vi "CWConvolution.vi"(0 "delay waveform":dbl[](array[numeric])=[0.0] format="%.2f", 1 "Boolean":bool, 2 "delay pts":i32, 3 "h(r,t)":dbl[](array[numeric]) format="%.2f", 4 "Variables":T1={"Number of rings"=8, "sound spd (cm/s)"=150000, "z span (cm)"=8.0, "z steps"=20, "y span (cm)"=0.2, "y steps"=20, "time step (s)"=1e-08, "z"=0.0, "y"=0.0, "ref delay"=0.0, "freq (MHz)"=4.71, "cycles"=300} {"freq (MHz)" format="%.2f"; "z span (cm)" format="%.2f"; "y" format="%.2f"; "ref delay" format="%.2f"; "y span (cm)" format="%.3f"; "z" format="%.2f"; "time step (s)" format="%.2e"}) -> (5 "X*Y":dbl[](array[numeric]) format="%.2f", 7 "pre-zeros":i32)   [LabVIEW 2022 SP3]
uses:
  <vilib>/Analysis/2dsp.llb/Real FFT.vi
  <vilib>/Analysis/2dsp.llb/Inverse Complex FFT.vi
  <vilib>/Analysis/2dsp.llb/1D Convolution (DBL).vi
  <vilib>/measure/NI_MABase.lvlib
  <vilib>/Analysis/NI_AALPro.lvlib
panel:
  in  "Case Constant\n(See Context Help)":bool
  out "Waveform Graph 2":dbl[](graph)
  out "Waveform Graph":dbl[](graph)
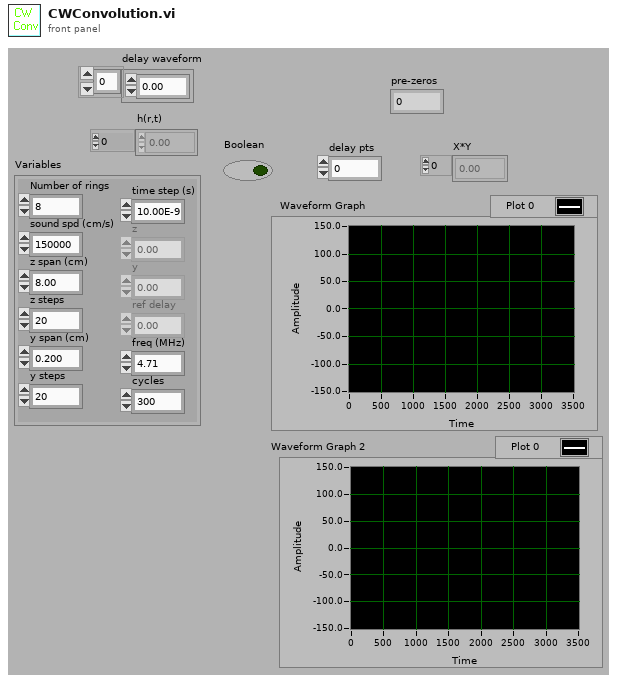
[diagram p1: front panel]
types:
  T1 = cluster{"Number of rings":i32, "sound spd (cm/s)":i32, "z span (cm)":dbl, "z steps":i32, "y span (cm)":dbl, "y steps":i32, "time step (s)":sgl, "z":dbl, "y":dbl, "ref delay":dbl, "freq (MHz)":dbl, "cycles":i32}
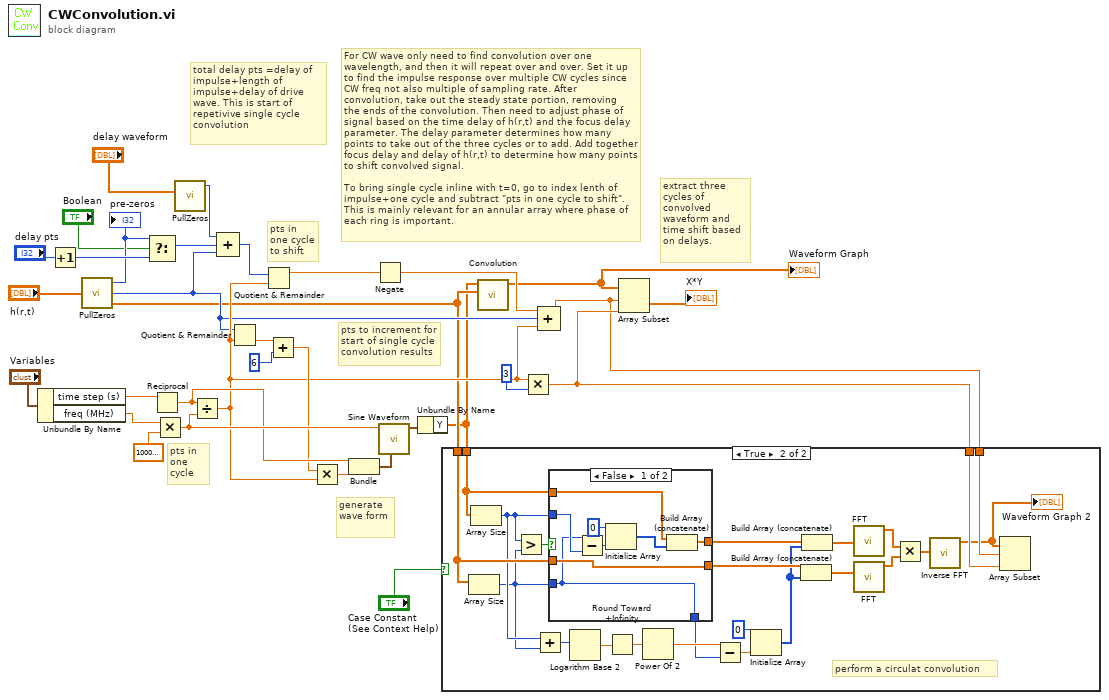
[diagram p0: block diagram]
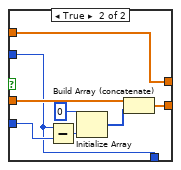
[diagram p3: hidden frame]
diagram:
  # "pts to increment for start of single cycle convolution results"
  # "extract three cycles of convolved waveform and time shift based on delays."
  # "generate wave form"
  # "pts in one cycle"
  # "pts in one cycle to shift"
  # "total delay pts =delay of impulse+length of impulse+delay of drive wave. This is start of repetivive single cycle convolution"
  # "For CW wave only need to find convolution over one wavelength, and then it will repeat over and over. Set it up to find the impulse response over multiple CW cycles since CW freq not also multiple of sampling rate. After convolution, take out the steady state portion, removing  the ends of the convolution. Then need to adjust phase of signal based on the time delay of h(r,t) and the focus delay parameter. The delay parameter determines how many points to take out of the three cycles or to add. Add together focus delay and delay of h(r,t) to determine how many points to shift convolved signal.\n\nTo bring single cycle inline with t=0, go to index lenth of impulse+one cycle and subtract \"pts in one cycle to shift\". This is mainly relevant for an annular array where phase of each ring is important."
  n1 = Unbundle By Name("Variables") -> ("time step (s)"=w22:sgl, "freq (MHz)"=w31:dbl)
  n2 = Increment(x="delay pts") -> (x+1=w10:i32)
  n3 = call "PullZeros.vi"("input"="h(r,t)") -> ("output"=w7:dbl[], "non zero points"=w16:i32, "pre-zeros"=w9:i32)  [unwired: 2 out]
  "pre-zeros" <- w9
  n4 = Select(t=w9, s="Boolean", f=w10) -> (s? t:f=w13:i32)
  n5 = Reciprocal(x=w22) -> (1/x=w28:sgl)
  n6 = Multiply(x=w31, y=1000000.0) -> (x*y=w29:dbl)
  n7 = call "PullZeros.vi"("input"="delay waveform") -> ("pre-zeros"=w17:i32)  [unwired: 4 out]
  n8 = Divide(x=w28, y=w29) -> (x/y=w20:dbl)
  n9 = Compound Arithmetic op=ADD(w17, w13, w16) -> (w15:i32)
  n10 = Quotient & Remainder(x=w16, y=w20) -> (floor(x/y)=w21:dbl)  [unwired: 1 out]
  n11 = Quotient & Remainder(x=w15, y=w20) -> (x-y*floor(x/y)=w19:dbl)  [unwired: 1 out]
  n12 = Add(x=w21, y=6) -> (x+y=w25:dbl)
  n13 = Multiply(x=w25, y=w20) -> (x*y=w27:dbl)
  n14 = Bundle(w28, w27) -> (w32:cluster{sgl, dbl})  [unwired: 1 out]
  n15 = Negate(x=w19) -> (-x=w14:dbl)
  n16 = call <vilib>:"Sine Waveform.vi"("sampling info"=w32, "frequency"=w29) -> ("signal out"=w26:waveform(dbl))  [unwired: 5 in, 4 out]
  n17 = Unbundle By Name(w26) -> ("Y"=w6:dbl[])
  n18 = call-poly <vilib>:"Convolution.vi"("Y"=w7, "X"=w6) -> ("X * Y"=w2:dbl[])  [unwired: 1 in, 8 out]
  "Waveform Graph" <- w2
  n19 = Multiply(x=w20, y=3) -> (x*y=w5:dbl)
  n20 = Compound Arithmetic op=ADD(w14, w16, w20) -> (w4:dbl)
  n21 = case shown="True" "Case Constant\n(See Context Help)" {
    tunnel: w7 -> [_ w52]
    tunnel: w6 -> [_ w51]
    tunnel: w5 -> [_ w50]
    tunnel: w4 -> [_ w49]
    frame False {
    }
    frame True {
      # "perform a circulat convolution"
      n22 = Array Size(array=w52) -> (size(s)=w47:i32)
      n23 = Array Size(array=w51) -> (size(s)=w48:i32)
      n24 = Greater?(x=w48, y=w47) -> (0:w53:bool)
      n25 = Add(x=w48, y=w47) -> (x+y=w46:i32)
      n26 = case shown="False" w53 {
        tunnel: w48 -> [w60 w65]
        tunnel: w47 -> [w57 w72]
        tunnel: w52 -> [w58 w69]
        tunnel: [w58 w67] -> w41
        tunnel: w51 -> [w61 w66]
        tunnel: [w59 w66] -> w40
        tunnel: [w57 w65] -> w37
        frame False {
          n27 = Subtract(x=w57, y=w60) -> (x-y=w63:i32)
          n28 = Initialize Array(0, w63) -> (w62:i32[])
          n29 = Build Array (concatenate)(w61, w62) -> (w59:dbl[])
        }
        frame True {
          n30 = Subtract(x=w65, y=w72) -> (x-y=w70:i32)
          n31 = Initialize Array(0, w70) -> (w68:i32[])
          n32 = Build Array (concatenate)(w69, w68) -> (w67:dbl[])
        }
      }
      n33 = Logarithm Base 2(1:w46) -> (0:w45:dbl)
      n34 = Round Toward +Infinity(x=w45) -> (ceil(x): smallest int >= x=w44:dbl)
      n35 = Power Of 2(x=w44) -> (2^x=w38:dbl)
      n36 = Subtract(x=w38, y=w37) -> (x-y=w42:dbl)
      n37 = Initialize Array(0, w42) -> (w39:i32[])
      n38 = Build Array (concatenate)(w41, w39) -> (w35:dbl[])
      n39 = Build Array (concatenate)(w40, w39) -> (w36:dbl[])
      n40 = call-poly <vilib>:"FFT.vi"("X"=w36) -> ("FFT {X}"=w56:cdb[])  [unwired: 2 in, 8 out]
      n41 = call-poly <vilib>:"FFT.vi"("X"=w35) -> ("FFT {X}"=w55:cdb[])  [unwired: 2 in, 8 out]
      n42 = Multiply(x=w56, y=w55) -> (x*y=w54:cdb[])
      n43 = call-poly <vilib>:"Inverse FFT.vi"("FFT {X}"=w54) -> ("X"=w34:cdb[])  [unwired: 1 in, 9 out]
      "Waveform Graph 2" <- w34
      n44 = Array Subset(array=w34, index=w49, length=w50) -> ()  [unwired: 1 out]
    }
  }
  n45 = Array Subset(array=w2, index=w4, length=w5) -> (→"X*Y":dbl[])
